vi "Builder.Create.vi"(8 "error in (no error)":errorcluster, 9 "Build Durations Pointer":refnum<class "Memory.Pointer.U32.lvclass">, 10 "Framework Cache":refnum<class "DSF.Engine.Memory.Cache.Framework.lvclass">, 11 "Builder type":refnum<class "Builder.lvclass">) -> (0 "error out":errorcluster, 3 "Builder":refnum<class "Builder.lvclass">)   [LabVIEW 2016, in "DSF.Engine.lvlib" / "Builder.lvclass"]
uses:
  Builder.lvclass
  Cache/DSF.Engine.Memory.Cache.Framework.lvclass
  Submodules/Memory/Source/Classes/Standard Types/Memory.Pointer.U32.lvclass
  Interface/DSF.Engine.Interface.lvclass/DSF.Engine.Interface.ctl
  Builder.lvclass/Builder.ctl
  Interface/DSF.Engine.Interface.New.vi
  Interface/DSF.Engine.Interface.RT FIFO.Create.vi
  Interface/DSF.Engine.Interface.Set Command FIFO.vi
  Interface/DSF.Engine.Interface.Set Response FIFO.vi
  Interface/DSF.Engine.Interface.Builder.lvclass
  C:/Git/Sourcetree/DSF/Source/Engine/Classes/Interface/DSF.Engine.Interface.lvclass
  Status/Builder Status.lvclass
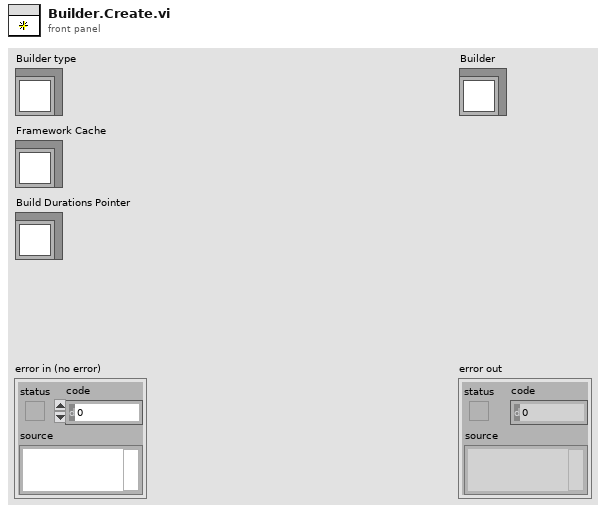
[diagram p1: front panel]
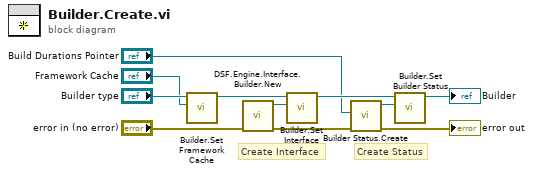
[diagram p0: block diagram]
diagram:
  # "Create Status"
  # "Create Interface"
  n1 = call "Builder.Set Framework Cache.vi"("Framework Cache"="Framework Cache", "Builder in"="Builder type") -> ("Builder out"=w1:refnum<class "Builder.lvclass">)  [unwired: 9 in]
  n2 = call "DSF.Engine.Interface.Builder.New.vi"("error in (no error)"="error in (no error)") -> ("error out"=w5:errorcluster, "Builder Interface"=w9:refnum<class "DSF.Engine.Interface.Builder.lvclass">)  [unwired: 9 in]
  n3 = call "Builder.Set Interface.vi"("Builder Interface"=w9, "Builder in"=w1) -> ("Builder out"=w7:refnum<class "Builder.lvclass">)  [unwired: 9 in]
  n4 = call "Builder Status.Create.vi"("error in (no error)"=w5, "Build Durations Pointer"="Build Durations Pointer") -> ("error out"=→"error out":errorcluster, "Builder Status"=w6:refnum<class "Builder Status.lvclass">)  [unwired: 8 in]
  n5 = call "Builder.Set Builder Status.vi"("Builder Status"=w6, "Builder in"=w7) -> ("Builder out"=→"Builder":refnum<class "Builder.lvclass">)  [unwired: 9 in]
